vi "emi_Set Application version from Containing VI.vi"(11 "error in (no error)":errorcluster) -> (15 "error out":errorcluster)   [LabVIEW 2010]
doc: "Set the application version information from the tags in witch it is placed.\n\n\nOn error. Try to get the version anyway.\nIf there is no user tag information: Return error"
uses:
  <vilib>/UserTags/UserTags.lvlib
  Private/emi_Version Info.ctl
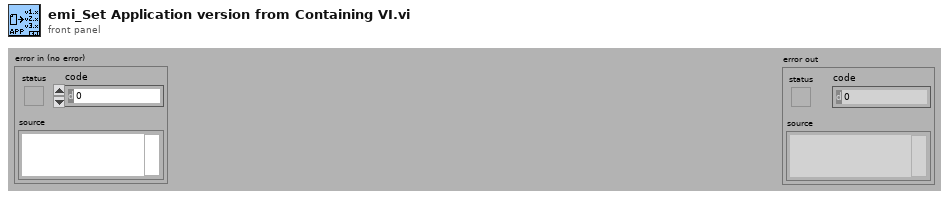
[diagram p1: front panel]
types:
  T1 = typedef "emi_Version Info.ctl" = cluster{"Name":string, "Major":i16, "Minor":i16, "Fix":i16, "Build":i32, "Type":enum16{"Alfa", "Beta", "Stable"}, "Dev":bool, "Version Name":string, "Date":timestamp}
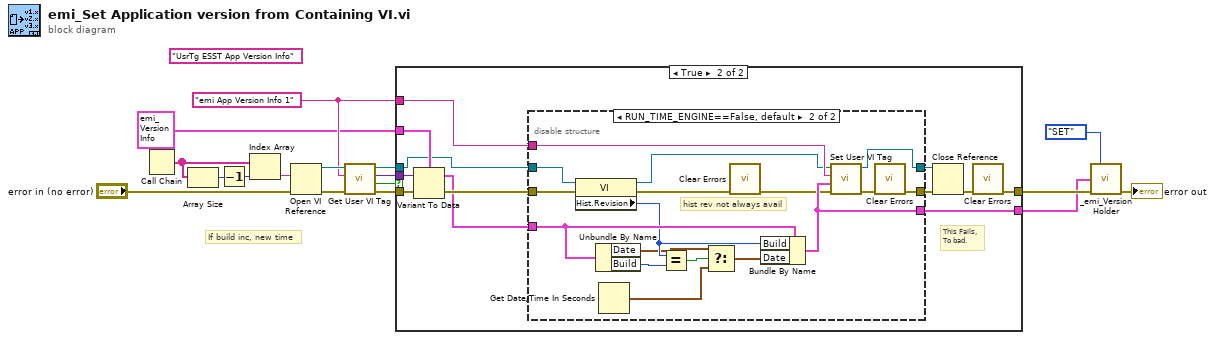
[diagram p0: block diagram]
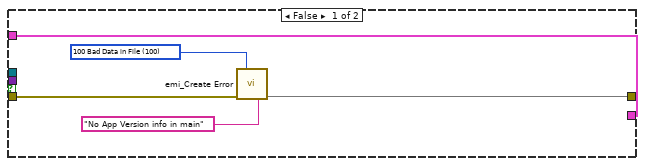
[diagram p2: hidden frame]
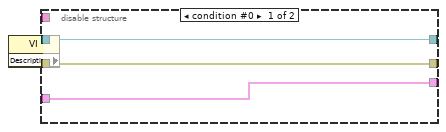
[diagram p3: hidden frame]
diagram:
  (unwired) "UsrTg ESST App Version Info" ("Tag Name")
  w6 = "emi App Version Info 1" ("Tag Name")
  # "If build inc, new time"
  n1 = Call Chain() -> (call chain=w14:string[])
  n2 = Array Size(array=w14) -> (size(s)=w15:i32)
  n3 = Decrement(x=w15) -> (x-1=w13:i32)
  n4 = Index Array(array=w14, index=w13) -> (element=w12:string)
  n5 = Open VI Reference(vi path=w12, error in (no error)="error in (no error)") -> (vi reference=w10:refnum<vi>, error out=w11:errorcluster)  [unwired: 4 out]
  n6 = call <vilib>:"Get User VI Tag.vi"("error in (no error)"=w11, "Tag Name"=w6, "VI Refnum"=w10) -> ("error out"=w9:errorcluster, "Was Tag Found?"=w1:bool, "Value"=w8:variant, "dup VI Refnum"=w7:refnum<vi>)  [unwired: 5 in]
  n7 = case shown="True" w1 {
    tunnel: w9 -> [w21 w32]
    tunnel: w8 -> [_ w31]
    tunnel: w7 -> [_ w23]
    tunnel: w6 -> [_ w28]
    tunnel: T1 {"Name"="NA", "Major"=0, "Minor"=0, "Fix"=0, "Build"=0, "Type"=enum."Alfa", "Dev"=FALSE, "Version Name"="", "Date"=timestamp(0 s since 1904-01-01)} ("Version Info in") -> [w22 w26]
    tunnel: [w20 w25] -> w4
    tunnel: [w22 w24] -> w2
    frame False {
      w19 = 100 items=["0 No Error"=0, "1 Invalid input parameter"=1, "6 Generic file IO "=6, "7 File not Found"=7, "35 Generic Pring Error"=35, "37 Device not Found"=37, "39 Device Unit Error"=39, "40 Could fot Open Device"=40, "42 Generic Error"=42, "52 Unknown Message"=52, "98 Bad File type"=98, "99 Bad File Version"=99, "100 Bad Data in File"=100, "1018 Unspecefied Error"=1018, "1041 Incorrect Password"=1041, "1043 Feature not in this version"=1043, "1109 Unsuported Data type"=1109] ("Error Code")
      n8 = call "emi_Create Error.vi"("Error Code"=w19, 11:w21, "Append String(\"\")"="No App Version info in main" ("Append String(\"\")")) -> (15:w20)  [unwired: 11 in, 1 out]
    }
    frame True {
      # "This Fails,\nTo bad."
      n9 = Variant To Data(error in=w32, Variant=w31, type=w26) -> (error out=w30:errorcluster, data=w29:T1)
      n10 = disable-structure shown="RUN_TIME_ENGINE==False, default" {
        disable-tunnel: w23 -> [w38 w55]
        disable-tunnel: [w37 w42] -> w34
        disable-tunnel: w30 -> [w36 w54]
        disable-tunnel: [w36 w48] -> w33
        disable-tunnel: w29 -> [w35 w51]
        disable-tunnel: w28 -> [_ w49]
        disable-tunnel: [w35 w47] -> w24
        frame condition #0 {
          n11 = property class="VI" props=["Description"](reference=w38, error in=w36) -> (reference out=w37:refnum<vi>)  [unwired: 2 out]
        }
        frame condition #1 (active) {
          # "hist rev not always avail"
          n12 = property class="VI"(reference=w55, error in=w54) -> (reference out=w41:refnum<vi>, error out=w40:errorcluster, "Hist.Revision"=w45:u32)
          n13 = Unbundle By Name(w51) -> ("Date"=w44:timestamp, "Build"=w50:i32)
          n14 = Get Date/Time In Seconds() -> (seconds since 1Jan1904=w43:timestamp)
          n15 = Equal?(x=w45, y=w50) -> (x = y?=w53:bool)
          n16 = Select(t=w44, s=w53, f=w43) -> (s? t:f=w46:timestamp)
          n17 = call <vilib>:"Clear Errors.vi"("error in (no error)"=w40) -> ("error out"=w39:errorcluster)  [unwired: 6 in]
          n18 = Bundle By Name(cluster=w51, "Build"=w45, "Date"=w46) -> (w47:T1)
          n19 = call <vilib>:"Set User VI Tag.vi"("error in (no error)"=w39, "Value"=w47, "Tag Name"=w49, "VI Refnum"=w41) -> ("error out"=w52:errorcluster, "dup VI Refnum"=w42:refnum<vi>)  [unwired: 5 in, 1 out]
          n20 = call <vilib>:"Clear Errors.vi"("error in (no error)"=w52) -> ("error out"=w48:errorcluster)  [unwired: 6 in]
        }
      }
      n21 = Close Reference(reference=w34, error in (no error)=w33) -> (error out=w27:errorcluster)
      n22 = call <vilib>:"Clear Errors.vi"("error in (no error)"=w27) -> ("error out"=w25:errorcluster)  [unwired: 6 in]
    }
  }
  n23 = call "_emi_Version Holder.vi"("Action(GET)"=enum16{"GET", "SET"}."SET", "Version Info in"=w2, "error in (no error)"=w4) -> ("error out"=→"error out":errorcluster)  [unwired: 10 in, 2 out]
